vi "testGPS_UTC.vi"() -> ()   [LabVIEW 2010]
uses:
  <instrlib>/niSync/niSync.llb/niSync Initialize (IVI).vi
panel:
  out "sys-GPS":dbl
  out "sys time":timestamp
  out "time GPS":timestamp
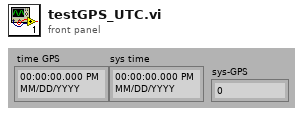
[diagram p1: front panel]
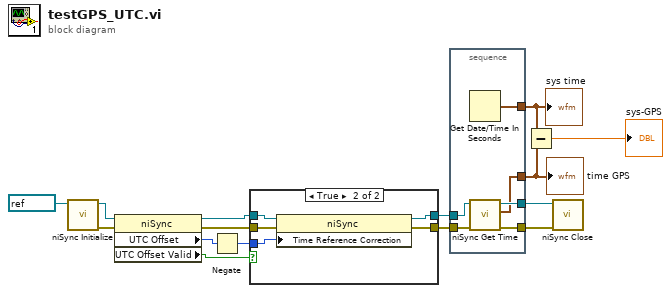
[diagram p0: block diagram]
diagram:
  n1 = call-poly <instrlib>:"niSync Initialize.vi"("resource name"=refnum<k15> "GPS") -> ("error out"=w13:errorcluster, "instrument handle out"=w14:refnum<k15>)  [unwired: 9 in]
  n2 = property class="niSync"(reference=w14, error in=w13) -> (reference out=w10:refnum<k15>, error out=w9:errorcluster, "UTC Offset"=w6:i32, "UTC Offset Valid"=w4:bool)
  n3 = Negate(x=w6) -> (-x=w5:i32)
  n4 = case shown="True" w4 {
    tunnel: w10 -> [w17 w22]
    tunnel: w9 -> [w16 w21]
    tunnel: [w17 w20] -> w8
    tunnel: [w16 w19] -> w7
    tunnel: w5 -> [_ w18]
    frame False {
    }
    frame True {
      n5 = property class="niSync"(reference=w22, error in=w21, "Time Reference Correction"=w18) -> (reference out=w20:refnum<k15>, error out=w19:errorcluster)
    }
  }
  n6 = stacked-sequence {
    tunnel: w8 -> [w28]
    tunnel: w7 -> [w27]
    tunnel: [w26] -> w12
    tunnel: [w25] -> w11
    tunnel: [w24] -> w2
    tunnel: [w23] -> w1
    frame #0 {
      n7 = Get Date/Time In Seconds() -> (seconds since 1Jan1904=w24:timestamp)
      n8 = call <instrlib>:"niSync Get Time.vi"("error in (no error)"=w27, "instrument handle"=w28) -> ("error out"=w25:errorcluster, "time"=w23:timestamp, "instrument handle out"=w26:refnum<k15>)  [unwired: 5 in]
    }
  }
  "sys time" <- w2
  "time GPS" <- w1
  n9 = Subtract(x=w2, y=w1) -> (x-y=→"sys-GPS":dbl)
  n10 = call <instrlib>:"niSync Close.vi"("error in (no error)"=w11, "instrument handle"=w12) -> ()  [unwired: 9 in, 1 out]
